vi "RT Driver VI.vi"(7 "Operation":T1, 11 "Device Reference in":T2 format="%.0x") -> (0 "Error Code":i32)   [LabVIEW 2017, in "Ballard MIL-1553 Engine.lvlib"]
uses:
  Ballard MIL-1553 Engine.lvlib
  <vilib>/NI Veristand/Custom Device API/Custom Device Item Ref.ctl
  <vilib>/NI Veristand/Custom Device API/Hardware Interface Driver VI Operation.ctl
  RT Driver/Controls/RT StateVariables.ctl
  <vilib>/NI/NIVS Inline Async API/_VS Inline Async API/VS Inline Async API/VS Inline Async API.lvclass
  RT Driver/Controls/Card Parameters.ctl
  Shared/Controls and Global/Initialization Method.ctl
  <vilib>/NI Veristand/Custom Device API/Data Reference.ctl
  RT Driver/Controls/RT Inline Data_Data Description_Channel.ctl
  RT Driver/Controls/RT Inline Frame Descriptor.ctl
  RT Driver/Controls/RT Inline Frame Descriptor_BC.ctl
  <vilib>/NI Veristand/Custom Device API/Block Data Reference.ctl
  RT Driver/Controls/RT Inline Frame Descriptor_RT.ctl
  Shared/Controls and Global/RT CWD2.ctl
  Shared/Controls and Global/RT CWD1.ctl
  Shared/Controls and Global/RT messageType.ctl
  RT Driver/Controls/RT Inline Broadcast Frame Descriptor.ctl
  RT Driver/Controls/Inline_Status_Channels.ctl
  <vilib>/NI/NIVS Inline Async API/_VS Inline Async API/VS Inline Async API/VS Inline Async API.lvclass/VS Inline Async API.ctl
  <vilib>/NI/NIVS Inline Async API/_Data Access Engine/Data Access Engine/Data Access Engine.lvclass/Data Access Engine.ctl
  <vilib>/NI/NIVS Inline Async API/_Data Access Engine/Access Type Classes/Write/Write.lvclass/Write.ctl
  <vilib>/NI/NIVS Inline Async API/_Data Access Engine/Access Type Classes/ReadWrite/ReadWrite.lvclass/ReadWrite.ctl
  <vilib>/NI/NIVS Inline Async API/_Data Access Engine/Access Type Classes/Read/Read.lvclass/Read.ctl
  <vilib>/NI/NIVS Inline Async API/_Data Access Engine/Data Access Engine/Methods/Data.Engine.Read Data from HW.vi
  <vilib>/NI/NIVS Inline Async API/_VS Inline Async API/Error Handling Process/SubVIs/Error.GetError.vi
  <vilib>/NI/NIVS Inline Async API/_Data Access Engine/Data Access Engine/Methods/Data.Engine.Write Data to HW.vi
  <vilib>/NI/NIVS Inline Async API/_Data Access Engine/Access Type Classes/ReadWrite/ReadWrite.EngineData.vi
  <vilib>/NI/NIVS Inline Async API/_Data Access Engine/Access Type Classes/Write/Write.EngineData.vi
  <vilib>/NI/NIVS Inline Async API/_Data Access Engine/Access Type Classes/Read/Read.EngineData.vi
  <vilib>/NI Veristand/Custom Device API/NI VeriStand - Get Channel Value by Data Reference.vi
  <vilib>/NI Veristand/Custom Device API/NI VeriStand - Set Channel Value by Data Reference.vi
  <vilib>/NI Veristand/Custom Device API/NI VeriStand - Get Channel Values by Block Data Reference.vi
  <vilib>/NI Veristand/Custom Device API/Global Data Refs.vi
  <vilib>/NI VeriStand/Custom Device Tools/Custom Device Utility Library/Custom Device Utility Library.lvlib
  Shared/Ballard 1553 Shared.lvlib
  <vilib>/NI VeriStand/Custom Device API/Custom Device API.lvlib
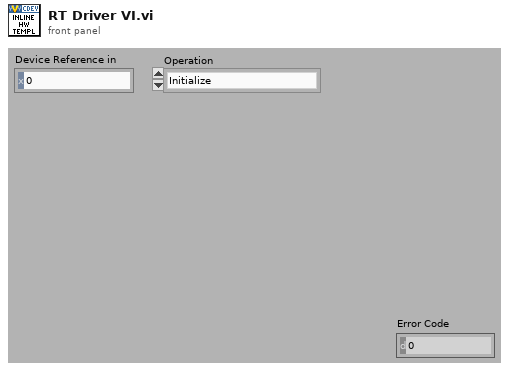
[diagram p1: front panel]
types:
  T1 = typedef "Custom Device API.lvlib/Hardware Interface Driver VI Operation.ctl" = enum16{"Initialize", "Start", "Read Data from HW", "Write Data to HW", "Close"}
  T2 = typedef "Custom Device API.lvlib/Custom Device Item Ref.ctl" = u64
  T3 = typedef "Ballard MIL-1553 Engine.lvlib/RT StateVariables.ctl" = cluster{"Async":refnum<class "VS Inline Async API.lvclass">, "Card Parameters (out)":T4, "Inline Status Channels Refs":T6[], "RT Inline Data_Data Description_Channels":T7[]}
  T4 = typedef "Ballard MIL-1553 Engine.lvlib/Card Parameters.ctl" = cluster{"card number":i32, "core number":i32, "core handle":u64, "core reader handle":u64, "channel handles[]":u64[], "Initialization Method":T5, "PXI slot number":i32}
  T5 = typedef "Ballard 1553 Shared.lvlib/Initialization Method.ctl" = enum16{"PXI Slot Number", "Card Number"}
  T6 = typedef "Custom Device API.lvlib/Data Reference.ctl" = i32
  T7 = typedef "Ballard MIL-1553 Engine.lvlib/RT Inline Data_Data Description_Channel.ctl" = cluster{"hardwareChannel":u16, "First Index for RT2RT Frames":i32, "Frame Drescriptors":T8[], "Broadcast Frame Descriptors":T15[]}
  T8 = typedef "Ballard MIL-1553 Engine.lvlib/RT Inline Frame Descriptor.ctl" = cluster{"BC":T9, "RT":T11, "Initialized?":bool, "RT to RT?":bool, "CWD2":T12, "CWD1":T13, "messageType":T14, "Name":string}
  T9 = typedef "Ballard MIL-1553 Engine.lvlib/RT Inline Frame Descriptor_BC.ctl" = cluster{"Timestamp?":bool, "Timestamp Channel Data Reference":T6, "Data Words?":bool, "Words Block Data Refs":T10[], "Sw1?":bool, "Sw2?":bool, "Status Channel Refs":T2[]}
  T10 = typedef "Custom Device API.lvlib/Block Data Reference.ctl" = cluster{"Data Reference":T6, "Offset":u64, "Length":u64}
  T11 = typedef "Ballard MIL-1553 Engine.lvlib/RT Inline Frame Descriptor_RT.ctl" = cluster{"Timestamp?":bool, "Timestamp Channel Data Reference":T6, "Data Words?":bool, "Words Block Data Refs":T10[], "Status Channel Ref?":bool, "Status Channel Ref":T2}
  T12 = typedef "Ballard 1553 Shared.lvlib/RT CWD2.ctl" = cluster{"TA (RT)":i8, "SA":i8, "Words (WC)":i8}
  T13 = typedef "Ballard 1553 Shared.lvlib/RT CWD1.ctl" = cluster{"TA (RT)":i8, "SA":i8, "Mode Code":i8, "Words Count":i8}
  T14 = typedef "Ballard 1553 Shared.lvlib/RT messageType.ctl" = enum16{"BC to RT", "RT to BC", "RT to RT", "MC (Rx)", "MC (Tx)"}
  T15 = typedef "Ballard MIL-1553 Engine.lvlib/RT Inline Broadcast Frame Descriptor.ctl" = cluster{"BC":T9, "Initialized?":bool, "RT to RT?":bool, "CWD2":T12, "CWD1":T13, "messageType":T14, "Name":string, "RTs":T11[]}
  T16 = typedef "Ballard MIL-1553 Engine.lvlib/Inline_Status_Channels.ctl" = enum16{"Error Code", "Inline Read Time (us)", "Inline Write Time (us)", "Unconfigured Frames Counter", "Monitor - Error Counter", "General Protocol Error Counter", "Wrong Sync Error Counter", "Improper Number of Data Words Error", "Manchester Error Counter", "Parity Error Counter", "Word Error Counter"}
  T17 = typedef "Ballard MIL-1553 Engine.lvlib/RT Async Data.ctl" = cluster{"Map (BC to RT)":T18[], "Raw Values (BC to RT)":T20, "Map (RT to ..)":T22[], "Raw Values (RT to ..)":T20, "Map (RTs Status)":T23[], "Raw Values (RTs Status)":T20, "Map (Bc Command Channels)":T24[], "MAP (BC Acyclic Messages Trigger)":T25[], "Map (RT Command Channels)":T26[], "Map (MC Rx)":T18[], "Raw Values (MC Rx)":T20, "Raw Values (MC Tx)":T20, "Map (MC Tx)":T22[]}
  T18 = typedef "Ballard MIL-1553 Engine.lvlib/RT Async_Map BC2RT.ctl" = cluster{"Channel Index":i32, "ID":i32, "Channel Data Reference":T6, "Word Index":i32, "Message Handle":u64, "Type":T19, "Word Count":i32, "First Element Index":i32}
  T19 = typedef "Ballard MIL-1553 Engine.lvlib/RT Async_Map_Type.ctl" = enum16{"Word (BC to RT)", "Word (MC (Rx))", "Acyclic Message Trigger", "Word (RT to ..)", "Word (RT to RT)", "Word (MC (Tx))", "RT Status", "BC Commands", "RT Commands"}
  T20 = typedef "Ballard MIL-1553 Engine.lvlib/RT Async_Raw Values.ctl" = cluster{"Association":T21[], "Raw Values Array":u16[]}
  T21 = typedef "Ballard MIL-1553 Engine.lvlib/RT Async_Raw Values to Messages Index_Association.ctl" = cluster{"Message Index":i32, "Raw Value Index":i32}
  T22 = typedef "Ballard MIL-1553 Engine.lvlib/RT Async_Map RT2BC.ctl" = cluster{"Channel Index":i32, "ID":i32, "Word Data Reference":T6, "First element Index":i32, "rt Transfer Handle":u64, "Type":T19, "Word Count":i32}
  T23 = typedef "Ballard MIL-1553 Engine.lvlib/RT Async_Map RTs Status.ctl" = cluster{"Channel Index":i32, "ID":i32, "rt Transfer Handle":u64, "Type":T19}
  T24 = typedef "Ballard MIL-1553 Engine.lvlib/RT Async_Map BC Command Channels.ctl" = cluster{"Channel Index":i32, "ID":i32, "BC Handle":u64, "Type":T19, "BC Command Channel Ref":T2, "Command Type":enum16{"Start Command", "Stop Command"}}
  T25 = typedef "Ballard MIL-1553 Engine.lvlib/RT Async_Map BC Acyclic Messages Trigger.ctl" = cluster{"Channel Index":i32, "BC Handle":u64, "Type":T19, "Acyclic Message Trigger Channel Ref":T2, "Message Name":string}
  T26 = typedef "Ballard MIL-1553 Engine.lvlib/RT Async_Map RT Command Channels.ctl" = cluster{"Channel Index":i32, "ID":i32, "RT Handle":u64, "Type":T19, "RT Command Channel Ref":T2, "Command Type":enum16{"Start Command", "Stop Command"}}
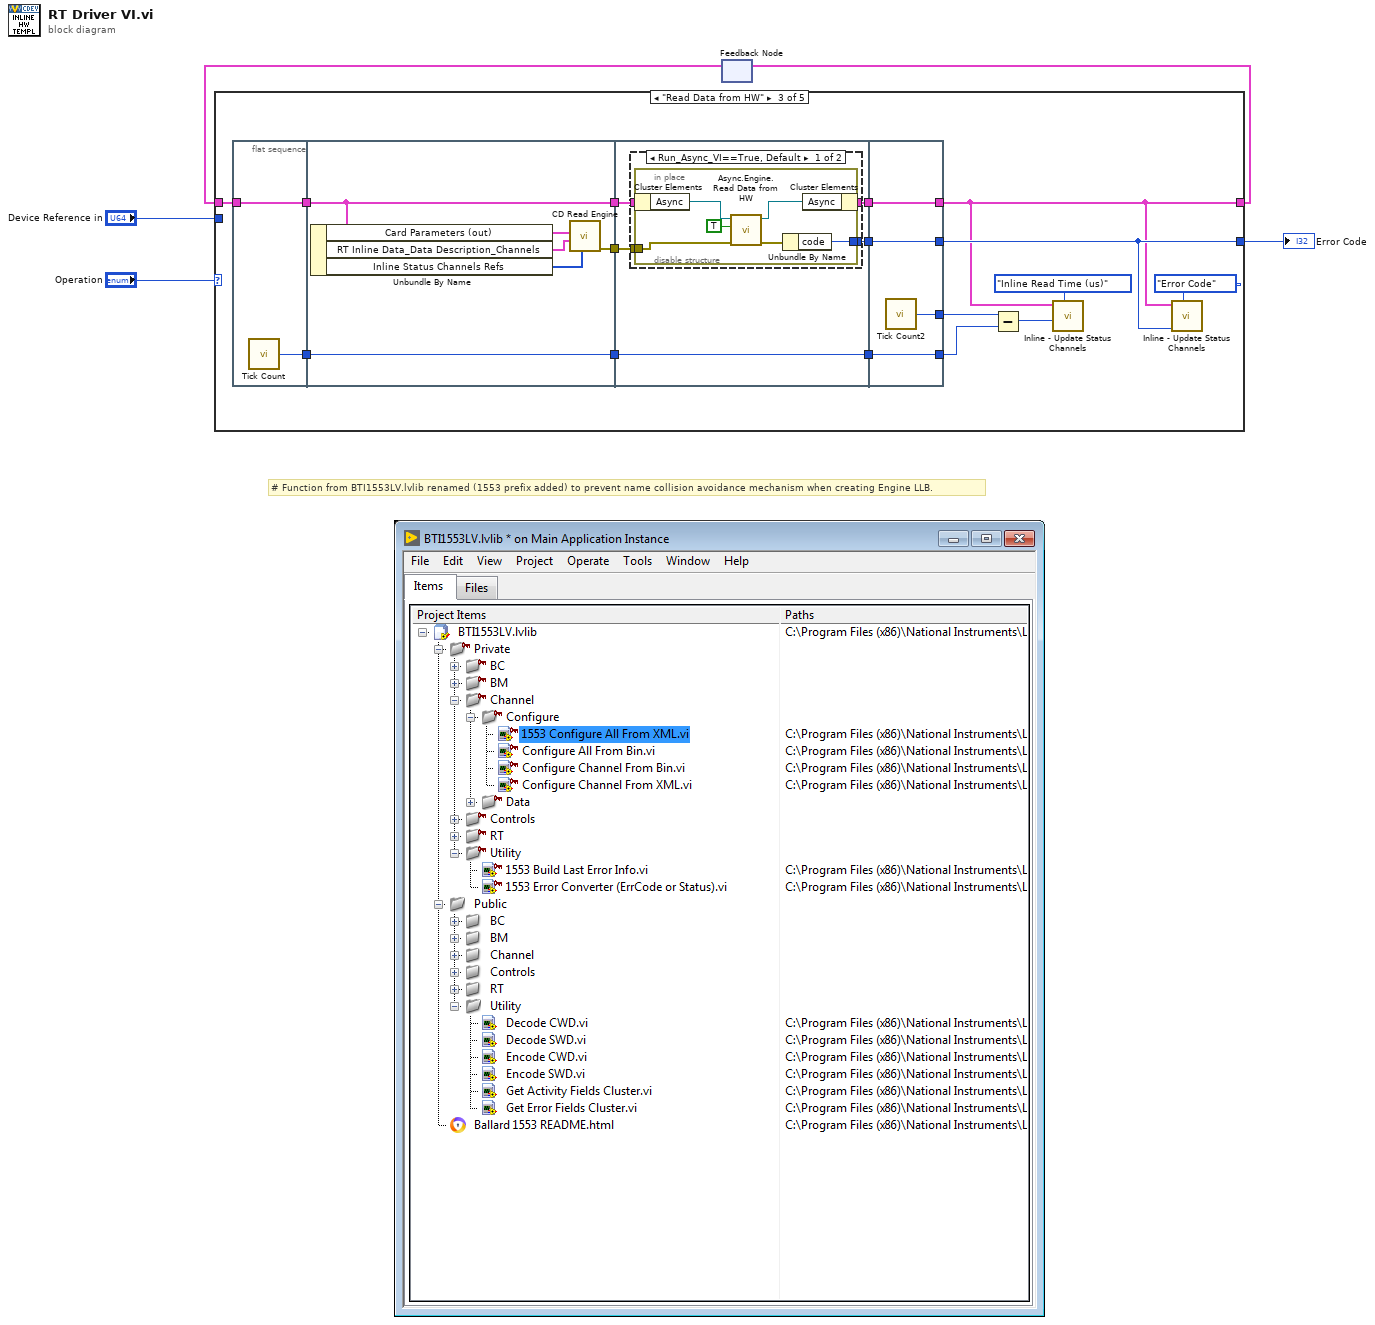
[diagram p0: block diagram]
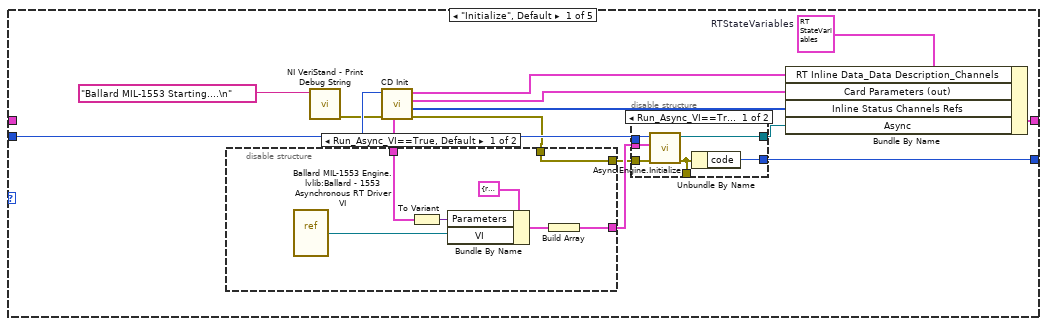
[diagram p2: hidden frame]
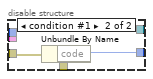
[diagram p4: hidden frame]
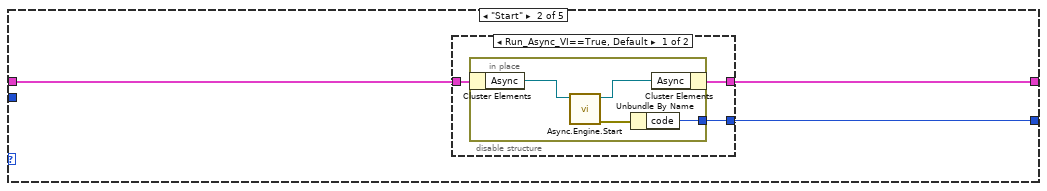
[diagram p5: hidden frame]
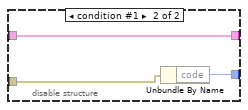
[diagram p7: hidden frame]
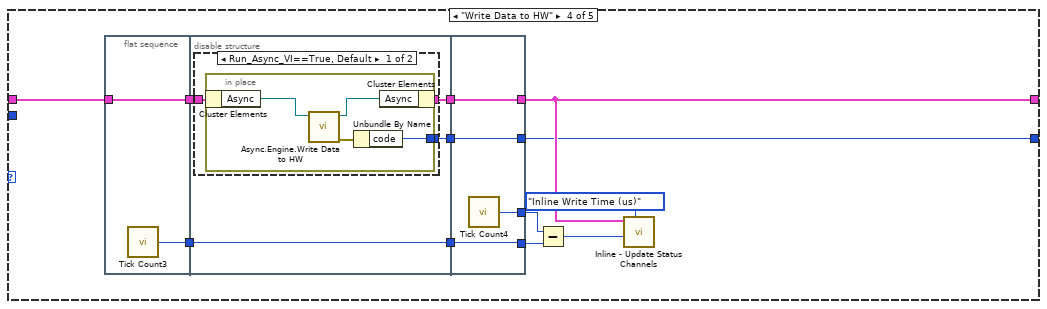
[diagram p8: hidden frame]
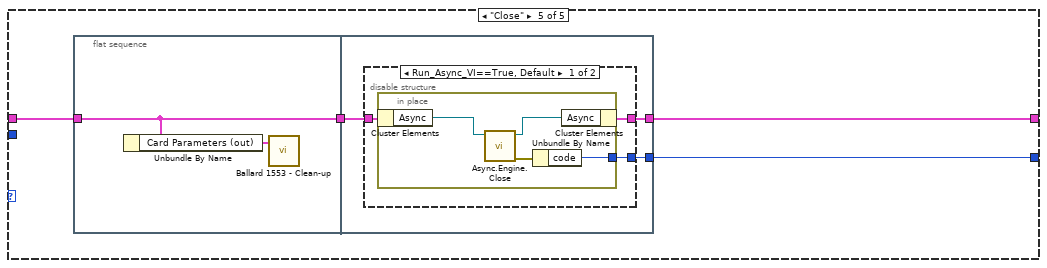
[diagram p10: hidden frame]
diagram:
  # "# Function from BTI1553LV.lvlib renamed (1553 prefix added) to prevent name collision avoidance mechanism when creating Engine LLB."
  n1 = feedback #1() -> (w4:T3)  [unwired: 1 out]
  n2 = case shown="\"Read Data from HW\"" "Operation" {
    tunnel: [w18 w38 w54 w95 w125] -> w5
    tunnel: w4 -> [_ w36 w62 w104 w126]
    tunnel: "Device Reference in" -> [w14 _ _ _ _]
    tunnel: [w8 w37 w57 w93 w124] -> w1
    frame "Initialize", Default {
      w17 = T3 {"Async"=refnum, "Card Parameters (out)"={"card number"=0, "core number"=0, "core handle"=0, "core reader handle"=0, "channel handles[]"=[], "Initialization Method"=enum."PXI Slot Number", "PXI slot number"=0}, "Inline Status Channels Refs"=[], "RT Inline Data_Data Description_Channels"=[]}  # RTStateVariables
      n3 = call <vilib>:"NI VeriStand - Print Debug String.vi"("Message"="Ballard MIL-1553 Starting....\n") -> ("error out"=w7:errorcluster)  [unwired: 10 in]
      n4 = call "CD Init.vi"("Error (in)"=w7, "Device Reference"=w14) -> ("Error (out)"=w9:errorcluster, "Inline Status Channels Refs"=w11:T6[], "Card Parameters (out)"=w12:T4, "RT Inline Data_Data Description_Channels"=w13:T7[], "RT Async Data"=w10:T17)  [unwired: 5 in]
      n5 = disable-structure shown="Run_Async_VI==True, Default" {
        disable-tunnel: [w24 _] -> w16
        disable-tunnel: w10 -> [w22 _]
        disable-tunnel: w9 -> [w21 w27]
        disable-tunnel: [w21 w27] -> w6
        frame condition #0 (active) {
          n6 = vi-ref "Ballard MIL-1553 Engine.lvlib:Ballard - 1553 Asynchronous RT Driver VI.vi"() -> (w20:refnum<vi>)
          n7 = To Variant(anything=w22) -> (Variant=w23:variant)
          n8 = Bundle By Name(cluster=cluster{"VI":refnum<vi>, "Parameters":variant} {"VI"=refnum, "Parameters"=variant} ("Process"), "Parameters"=w23, "VI"=w20) -> (w25:cluster{"VI":refnum<vi>, "Parameters":variant})
          n9 = Build Array(w25) -> (w24:cluster{"VI":refnum<vi>, "Parameters":variant}[])
        }
        frame condition #1 {
        }
      }
      n10 = disable-structure shown="Run_Async_VI==True, Default" {
        disable-tunnel: [w33 w34] -> w8
        disable-tunnel: [w32 _] -> w19
        disable-tunnel: w16 -> [w31 _]
        disable-tunnel: w6 -> [w30 w35]
        disable-tunnel: w14 -> [w29 _]
        disable-tunnel: [w28 _] -> _
        frame condition #0 (active) {
          n11 = call <vilib>:"Async.Engine.Initialize.vi"("error in (no error)"=w30, "Processes"=w31, "Custom Device Ref"=w29) -> ("error out"=w28:errorcluster, "Async"=w32:refnum<class "VS Inline Async API.lvclass">)  [unwired: 7 in]
          n12 = Unbundle By Name(w28) -> ("code"=w33:i32)
        }
        frame condition #1 {
          n13 = Unbundle By Name(w35) -> ("code"=w34:i32)
        }
      }
      n14 = Bundle By Name(cluster=w17, "RT Inline Data_Data Description_Channels"=w13, "Card Parameters (out)"=w12, "Inline Status Channels Refs"=w11, "Async"=w19) -> (w18:T3)
    }
    frame "Start" {
      n15 = disable-structure shown="Run_Async_VI==True, Default" {
        disable-tunnel: w36 -> [w41 w46]
        disable-tunnel: [w40 w46] -> w38
        disable-tunnel: [w39 _] -> w37
        frame condition #0 (active) {
          n16 = in-place {
            in-place-border: [w42] -> w39
            n17 = in-place-cluster #2(w41) -> ("Async"=w45:refnum<class "VS Inline Async API.lvclass">)
            n18 = call <vilib>:"Async.Engine.Start.vi"("VS Inline Async API in"=w45) -> ("error out"=w43:errorcluster, "VS Inline Async API out"=w44:refnum<class "VS Inline Async API.lvclass">)  [unwired: 9 in]
            n19 = Unbundle By Name(w43) -> ("code"=w42:i32)
            n20 = in-place-cluster #2("Async"=w44) -> (w40:T3)
          }
        }
        frame condition #1 {
        }
      }
    }
    frame "Read Data from HW" {
      n21 = flat-sequence {
        tunnel: w62 -> [w64]
        tunnel: [w64] -> w61
        tunnel: [w63] -> w60
        tunnel: [w69] -> w53
        tunnel: [w70] -> w51
        tunnel: w60 -> [w70]
        tunnel: w61 -> [w69]
        tunnel: [w65] -> w48
        tunnel: w53 -> [w74]
        tunnel: [w73] -> w52
        tunnel: w51 -> [w75]
        tunnel: [w75] -> w50
        tunnel: [w71] -> w49
        tunnel: w48 -> [w72]
        tunnel: [w91] -> w54
        tunnel: [w92] -> w57
        tunnel: w52 -> [w91]
        tunnel: [w90] -> w59
        tunnel: w50 -> [w89]
        tunnel: [w89] -> w58
        tunnel: w49 -> [w92]
        frame #0 {
          n22 = call "Tick Count"() -> ("Tick Count(uSec)"=w63:u32)
        }
        frame #1 {
          n23 = Unbundle By Name(w69) -> ("Card Parameters (out)"=w68:T4, "RT Inline Data_Data Description_Channels"=w66:T7[], "Inline Status Channels Refs"=w67:T6[])
          n24 = call "CD Read Engine.vi"("Inline Status Channels Refs"=w67, "RT Inline Data_Data Description_Channels"=w66, "Card Parameters (in)"=w68) -> ("Error (out)"=w65:errorcluster)  [unwired: 6 in, 1 out]
        }
        frame #2 {
          n25 = disable-structure shown="Run_Async_VI==True, Default" {
            disable-tunnel: [w79 w86] -> w71
            disable-tunnel: w74 -> [w78 w88]
            disable-tunnel: [w77 w88] -> w73
            disable-tunnel: w72 -> [w76 w87]
            frame condition #0 (active) {
              n26 = in-place {
                in-place-border: [w83] -> w79
                in-place-border: w76 -> [w80]
                n27 = in-place-cluster #3(w78) -> ("Async"=w85:refnum<class "VS Inline Async API.lvclass">)
                n28 = call <vilib>:"Async.Engine.Read Data from HW.vi"("error in"=w80, "Report Error to Inline?"=TRUE, "Async in"=w85) -> ("error out"=w82:errorcluster, "Async out"=w84:refnum<class "VS Inline Async API.lvclass">)  [unwired: 7 in]
                n29 = Unbundle By Name(w82) -> ("code"=w83:i32)
                n30 = in-place-cluster #3("Async"=w84) -> (w77:T3)
              }
            }
            frame condition #1 {
              n31 = Unbundle By Name(w87) -> ("code"=w86:i32)
            }
          }
        }
        frame #3 {
          n32 = call "Tick Count2"() -> ("Tick Count(uSec)"=w90:u32)
        }
      }
      n33 = Subtract(x=w59, y=w58) -> (x-y=w55:u32)
      n34 = call "Inline - Update Status Channels.vi"("Status Channel"=Inline_Status_Channels."Inline Read Time (us)", "Time (us)"=w55, "RTStateVariables"=w54) -> ()  [unwired: 9 in]
      n35 = call "Inline - Update Status Channels.vi"("Status Channel"=Inline_Status_Channels."Error Code", "Error Code"=w57, "RTStateVariables"=w54) -> ()  [unwired: 9 in]
    }
    frame "Write Data to HW" {
      n36 = flat-sequence {
        tunnel: w104 -> [w106]
        tunnel: [w106] -> w103
        tunnel: [w105] -> w100
        tunnel: w103 -> [w107]
        tunnel: [w110] -> w102
        tunnel: [w109] -> w101
        tunnel: w100 -> [w108]
        tunnel: [w108] -> w99
        tunnel: [w121] -> w95
        tunnel: [w122] -> w93
        tunnel: w102 -> [w122]
        tunnel: w101 -> [w121]
        tunnel: [w120] -> w97
        tunnel: w99 -> [w119]
        tunnel: [w119] -> w98
        frame #0 {
          n37 = call "Tick Count3"() -> ("Tick Count(uSec)"=w105:u32)
        }
        frame #1 {
          n38 = disable-structure shown="Run_Async_VI==True, Default" {
            disable-tunnel: [w113 _] -> w110
            disable-tunnel: w107 -> [w112 w118]
            disable-tunnel: [w111 w118] -> w109
            frame condition #0 (active) {
              n39 = in-place {
                in-place-border: [w117] -> w113
                n40 = in-place-cluster #4(w112) -> ("Async"=w115:refnum<class "VS Inline Async API.lvclass">)
                n41 = call <vilib>:"Async.Engine.Write Data to HW.vi"("VS Inline Async API in"=w115) -> ("error out"=w116:errorcluster, "VS Inline Async API out"=w114:refnum<class "VS Inline Async API.lvclass">)  [unwired: 9 in]
                n42 = Unbundle By Name(w116) -> ("code"=w117:i32)
                n43 = in-place-cluster #4("Async"=w114) -> (w111:T3)
              }
            }
            frame condition #1 {
            }
          }
        }
        frame #2 {
          n44 = call "Tick Count4"() -> ("Tick Count(uSec)"=w120:u32)
        }
      }
      n45 = Subtract(x=w97, y=w98) -> (x-y=w96:u32)
      n46 = call "Inline - Update Status Channels.vi"("Status Channel"=Inline_Status_Channels."Inline Write Time (us)", "Time (us)"=w96, "RTStateVariables"=w95) -> ()  [unwired: 9 in]
    }
    frame "Close" {
      n47 = flat-sequence {
        tunnel: w126 -> [w128]
        tunnel: [w128] -> w123
        tunnel: [w130] -> w125
        tunnel: [w129] -> w124
        tunnel: w123 -> [w131]
        frame #0 {
          n48 = Unbundle By Name(w128) -> ("Card Parameters (out)"=w127:T4)
          n49 = call "Ballard 1553 - Clean-up.vi"("Card Parameters"=w127) -> ()  [unwired: 10 in, 1 out]
        }
        frame #1 {
          n50 = disable-structure shown="Run_Async_VI==True, Default" {
            disable-tunnel: w131 -> [w134 w139]
            disable-tunnel: [w133 w139] -> w130
            disable-tunnel: [w132 _] -> w129
            frame condition #0 (active) {
              n51 = in-place {
                in-place-border: [w136] -> w132
                n52 = in-place-cluster #5(w134) -> ("Async"=w138:refnum<class "VS Inline Async API.lvclass">)
                n53 = call <vilib>:"Async.Engine.Close.vi"("Async in"=w138) -> ("error out"=w135:errorcluster, "Async out"=w137:refnum<class "VS Inline Async API.lvclass">)  [unwired: 9 in]
                n54 = Unbundle By Name(w135) -> ("code"=w136:i32)
                n55 = in-place-cluster #5("Async"=w137) -> (w133:T3)
              }
            }
            frame condition #1 {
            }
          }
        }
      }
    }
  }
  "Error Code" <- w1
  n56 = feedback-in #1(w5) -> ()
